vi "9093_第8回課題2.vi"() -> ()   [LabVIEW 2020]
panel:
  out "出力電流":fxp<+/-,64,32>
  out "出力回数":i32
  out "出力波形":dbl(graph)=-1.0269562977782698e-15
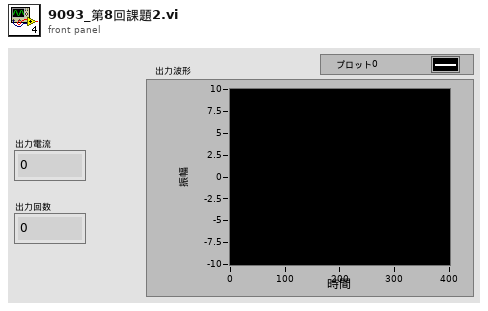
[diagram p1: front panel]
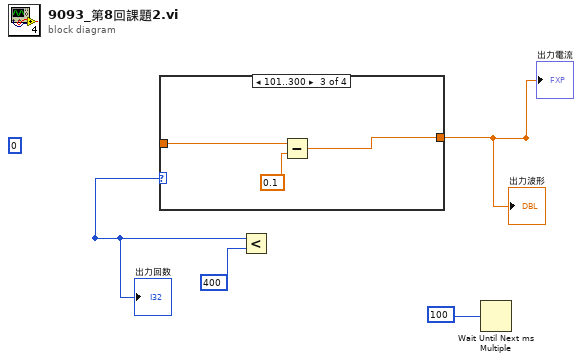
[diagram p0: block diagram]
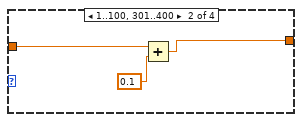
[diagram p3: hidden frame]
diagram:
  w7 = 0
  n1 = Less?(y=400) -> (x=w3:i32, x < y?=w4:bool)
  "出力回数" <- w3
  n2 = case shown="101..300" w3 {
    tunnel: [w8 w9 w14 w15] -> w1
    tunnel: [w8 w10 w13 w15] -> w2
    frame 0 {
    }
    frame 1..100, 301..400 {
      n3 = Add(x=w10, y=0.1) -> (x+y=w9:dbl)
    }
    frame 101..300 {
      n4 = Subtract(x=w13, y=0.1) -> (x-y=w14:dbl)
    }
    frame Default {
    }
  }
  "出力波形" <- w1
  "出力電流" <- w1
  n5 = Wait Until Next ms Multiple(millisecond multiple=100) -> ()  [unwired: 1 out]
